vi "Max compressed size.vi"(8 "error in (no error)":errorcluster, 10 "source size (bytes)":i32) -> (0 "error out":errorcluster, 2 "maximum compressed size (bytes)":i32)   [LabVIEW 2020, in "lvzstd.lvlib"]
uses:
  lvzstd.lvlib
  Private/Path FGV.vi
  <vilib>/Utility/error.llb/Error Cluster From Error Code.vi
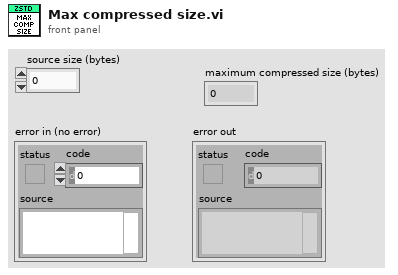
[diagram p1: front panel]
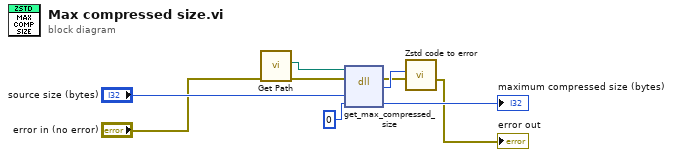
[diagram p0: block diagram]
diagram:
  n1 = call "Get Path.vi"("error in (no error)"="error in (no error)") -> ("error out (no error)"=w5:errorcluster, "Library Path"=w4:path)  [unwired: 9 in]
  n2 = dll-call lib="?" fn="get_max_compressed_size"(path in=w4, error in=w5, "source_size"="source size (bytes)", "max_compressed_size"=0) -> (error out=w2:errorcluster, "return type"=w3:i32, "max_compressed_size"=→"maximum compressed size (bytes)":i32)  [unwired: 2 in, 1 out]
  n3 = call "Zstd code to error.vi"("error in"=w2, "Error code"=w3) -> ("error in (no error)"=→"error out":errorcluster)  [unwired: 9 in]
